vi "Day7_Dashboard.vi"() -> ()   [LabVIEW 2025]
uses:
  <vilib>/Platform/TimedLoop/XDataNode/timing_clust.ctl
  <vilib>/Platform/TimedLoop/XDataNode/nitl_modes.ctl
  <vilib>/Platform/TimedLoop/XDataNode/wakeup.ctl
  <vilib>/Utility/error.llb/Trim Whitespace One-Sided.vi
  <vilib>/Instr/_visa.llb/VISA Configure Serial Port (Instr).vi
  <vilib>/Utility/file.llb/Write Delimited Spreadsheet (DBL).vi
  <vilib>/platform/TimedLoop/XDataNode/XDataNode.xnode
  <vilib>/Platform/TimedLoop/XDataNode/XDNodeRunTimeDep.lvlib
  <vilib>/ptbypt/NI_PtbyPt.lvlib
panel:
  in  "Tab Control":enum32{"Live View", "Stats", "Test Results"}(tab)
  out "Session Time (s)":dbl
  out "Timestamp":dbl
  out "Hall Sensor":dbl
  out "Touch Pin":dbl
  out "ADC (mv)":dbl
  out "mean":dbl format="%0.2f"
  in  "stop":bool
  out "Std Dev":dbl
  out "Mean":dbl
  out "Min":dbl
  out "Max":dbl
  in  "Touch Hi Limit":dbl
  in  "Touch Lo Limit":dbl
  out "Touch PASS":bool
  out "Touch FAIL":bool
  in  "Log File Path":path
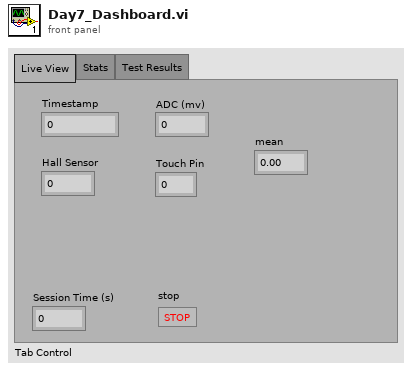
[diagram p1: front panel]
types:
  T1 = typedef "XDNodeRunTimeDep.lvlib/timing_clust.ctl" = cluster{"Expected End [f-1]":u64, "Actual End [f-1]":u64, "Finished Late? [f-1]":bool, "Expected End [i-1]":u64, "Actual End [i-1]":u64, "Finished Late? [i-1]":bool, "Expected Start [i]":u64, "Actual Start [i]":u64, "Expected Start [f]":u64, "Actual Start [f]":u64, "Source Name":string, "Structure Name":string, "Period":i64, "Deadline":i64, "Offset":i64, "Start":i64, "Priority":i32, "Timeout":i32, "Mode":T2, "Wakeup Reason":T3, "Error":errorcluster, "Source Type":string, "Secondary Source Type":string, "Global End Time":u64, "Global Start Time":u64, "Frame Duration":u64, "Iteration Duration":u64, "Assigned CPU":i32, "I/O Scan Engine Mode":u32}
  T2 = typedef "XDNodeRunTimeDep.lvlib/nitl_modes.ctl" = enum32{"No Change", "Process missed periods, maintain original phase", "Discard missed periods, maintain original phase", "Process missed periods, ignore original phase", "Discard missed periods, ignore original phase"}
  T3 = typedef "XDNodeRunTimeDep.lvlib/wakeup.ctl" = enum32{"Normal", "Aborted", "Asynchronous wakeup", "Timing source error", "Timed loop error", "Timeout"}
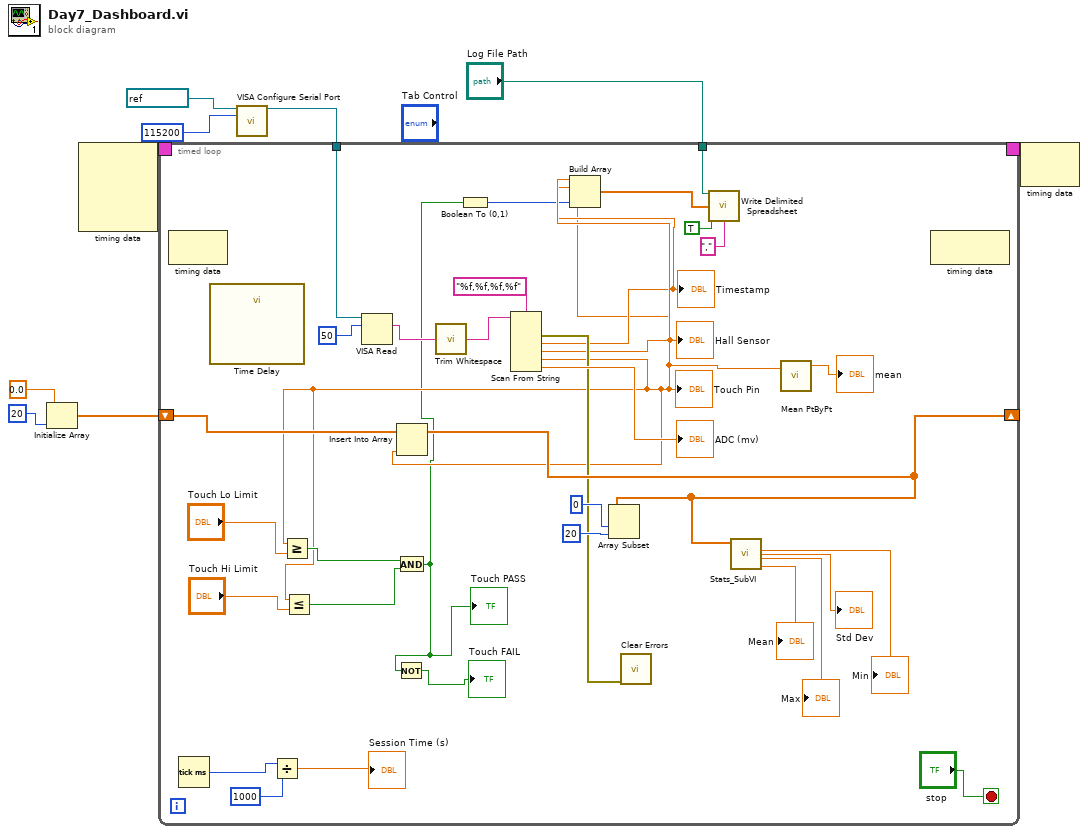
[diagram p0: block diagram]
diagram:
  n1 = Initialize Array "Initialize Array"(0.0 ("element"), 20 ("dimension size")) -> (w4:dbl[])
  n2 = node-c288() -> (w7:T1)  [unwired: 4 in]
  n3 = call-poly "VISA Configure Serial Port"("VISA resource name"=refnum<visa-resource-name> "COM4", "baud rate (9600)"=u32 115200) -> ("VISA resource name out"=w5:refnum<visa-resource-name>)  [unwired: 12 in, 1 out]
  n4 = timed-loop {
    timing: w7 -> [_]
    timing-out: [_] -> w6
    tunnel: w5 -> [w38]
    shift-right: [w32] -> _
    shift-left: w4 -> [w35]
    tunnel: "Log File Path" -> [w15]
    stop <- "stop" stop-if-true
    n5 = node-c288() -> ()  [unwired: 1 in, 1 out]
    n6 = Tick Count (ms)() -> (millisecond timer value=w12:u32)
    n7 = call "Time Delay"() -> ()  [unwired: 11 in, 1 out]
    n8 = Divide(x=w12, y=u32 1000) -> (x/y=→"Session Time (s)":dbl)
    n9 = VISA Read(VISA resource name=w38, byte count=u32 50) -> (read buffer=w42:string)  [unwired: 1 in, 3 out]
    n10 = call <vilib>:"Trim Whitespace.vi"("string"=w42) -> ("trimmed string"=w41:string)  [unwired: 1 in]
    n11 = Scan From String "Scan From String"(format string="%f,%f,%f,%f", input string=w41) -> (error out=w23:errorcluster, output 1=w19:dbl, output 2=w18:dbl, output 3=w21:dbl, output 4=→"ADC (mv)":dbl)  [unwired: 6 in, 2 out]
    "Timestamp" <- w19
    "Hall Sensor" <- w18
    "Touch Pin" <- w21
    n12 = Greater Or Equal?(x=w21, y="Touch Lo Limit") -> (x >= y?=w26:bool)
    n13 = Less Or Equal?(x=w21, y="Touch Hi Limit") -> (x <= y?=w25:bool)
    n14 = Insert Into Array "Insert Into Array"(array=w35, new element=w21) -> (w32:dbl[])  [unwired: 1 in]
    n15 = And(x=w26, y=w25) -> (x .and. y?=w17:bool)
    "Touch PASS" <- w17
    n16 = Not(x=w17) -> (.not. x?=→"Touch FAIL":bool)
    n17 = Boolean To (0,1)(Boolean=w17) -> (0, 1=w16:i16)
    n18 = Build Array "Build Array"(w21, w19, w18, w16) -> (w20:dbl[])
    n19 = Array Subset "Array Subset"(array=w32, index=0, length=20) -> ()  [unwired: 1 out]
    n20 = call <vilib>:"Clear Errors.vi"("error in (no error)"=w23) -> ()  [unwired: 5 in, 2 out]
    n21 = call-poly <vilib>:"Write Delimited Spreadsheet.vi"("file path (dialog if empty)"=w15, "1D data"=w20, "append to file? (new file:F)"=TRUE, "delimiter (\\t)"="," ("delimiter (\\t)")) -> ()  [unwired: 10 in, 2 out]
    n22 = call "Stats_SubVI.vi"("Input Array"=w32) -> ("Std Dev"=→"Std Dev":dbl, "Mean"=→"Mean":dbl, "Max"=→"Max":dbl, "Min"=→"Min":dbl)
    n23 = call <vilib>:"Mean PtByPt.vi"("x"=w21) -> ("mean"=→"mean":dbl)  [unwired: 3 in, 1 out]
    n24 = node-c288() -> ()  [unwired: 1 in, 1 out]
  }
  n25 = node-c288(w6) -> ()  [unwired: 1 out]
